vi "Close Config.vi"(8 "error in (no error)":errorcluster, 11 "Configuration File File In":refnum<class "Configuration File.lvclass">) -> (0 "error out":errorcluster, 3 "Configuration File File Out":refnum<class "Configuration File.lvclass">)   [LabVIEW 2020, in "Configuration File.lvclass"]
doc: "High-level function for opening configuration file data from Process class."
uses:
  Configuration File.lvclass
  C:/git/astemes-triarc-framework/source/Framework/Configuration/Configuration.lvclass
  Configuration/Protected/Get Config Ref.vi
  <vilib>/Utility/error.llb/Clear Errors.vi
  Base/Base.lvclass
  <vilib>/Utility/config.llb/NI_LVConfig.lvlib
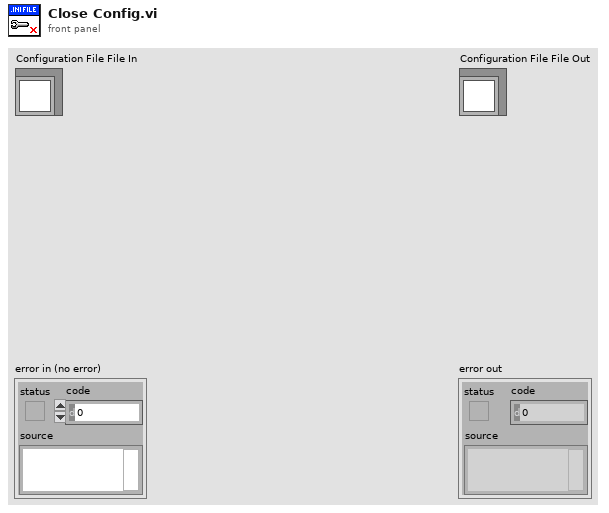
[diagram p1: front panel]
types:
  T1 = typedef "NI_LVConfig.lvlib/Config Data RefNum.ctl" = refnum<k1>
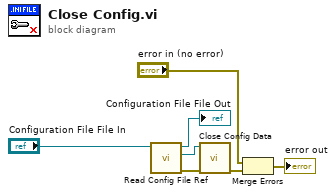
[diagram p0: block diagram]
diagram:
  n1 = call "Read Config File Ref.vi"("Configuration File In"="Configuration File File In") -> ("error out"=w7:errorcluster, "refnum out"=w3:T1, "Configuration File Out"=→"Configuration File File Out":refnum<class "Configuration File.lvclass">)  [unwired: 8 in]
  n2 = call <vilib>:"Close Config Data.vi"("error in (no error)"=w7, "refnum"=w3) -> ("error out"=w5:errorcluster)  [unwired: 8 in, 1 out]
  n3 = Merge Errors("error in (no error)", w5) -> (→"error out":errorcluster)
